vi "Search Project for XML Files.vi"(8 "error in (no error)":errorcluster, 11 "project reference":refnum<vi>) -> (0 "error out":errorcluster, 2 "xml files found":path[](array[path]))   [LabVIEW 2019, in "Configuration Tool.lvlib"]
uses:
  Configuration Tool.lvlib
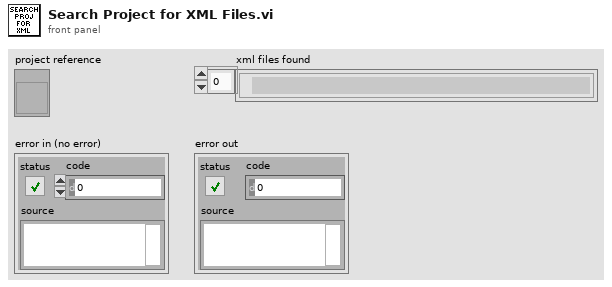
[diagram p1: front panel]
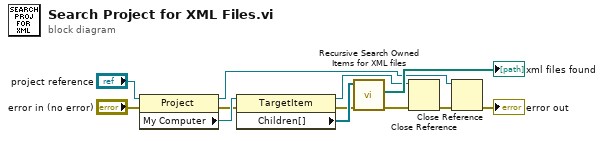
[diagram p0: block diagram]
diagram:
  n1 = property class="Project"(reference="project reference", error in="error in (no error)") -> (reference out=w3:refnum<vi>, error out=w7:errorcluster, "My Computer"=w11:refnum<vi>)
  n2 = property class="TargetItem"(reference=w11, error in=w7) -> (reference out=w5:refnum<vi>, error out=w6:errorcluster, "Children[]"=w10:refnum<vi>[])
  n3 = call "Recursive Search Owned Items for XML files.vi"("error in (no error)"=w6, "Owned Items[]"=w10) -> ("error out"=w2:errorcluster, "xml files found"=→"xml files found":path[])  [unwired: 8 in]
  n4 = Close Reference(reference=w5, error in (no error)=w2) -> (error out=w4:errorcluster)
  n5 = Close Reference(reference=w3, error in (no error)=w4) -> (error out=→"error out":errorcluster)
